vi "Write Sample Push.Sample mBar.vi"(6 "Publish (T)":bool=TRUE, 8 "error in (no error)":errorcluster, 10 "Sample mBar (0)":dbl, 11 "cRIO-CO2 in":refnum<class "cRIO-CO2.lvclass">) -> (0 "error out":errorcluster, 3 "cRIO-CO2 out":refnum<class "cRIO-CO2.lvclass">)   [LabVIEW 2015, in "cRIO-Carbondioxide.lvlib" / "cRIO-CO2.lvlib" / "cRIO-CO2.lvclass"]
uses:
  cRIO-CO2.lvclass
  cRIO-CO2.lvclass/cRIO-CO2.ctl
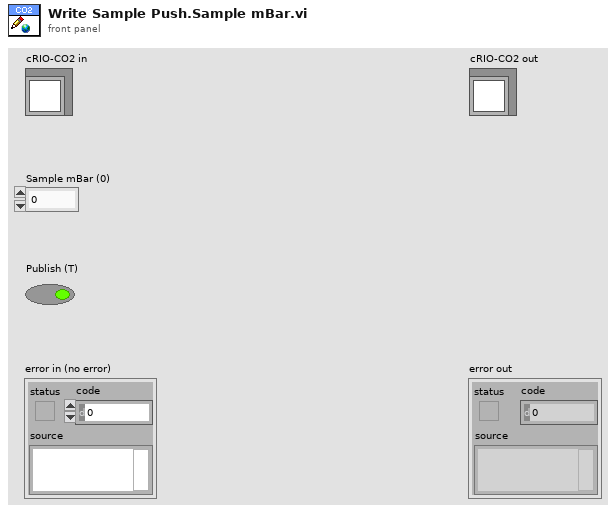
[diagram p1: front panel]
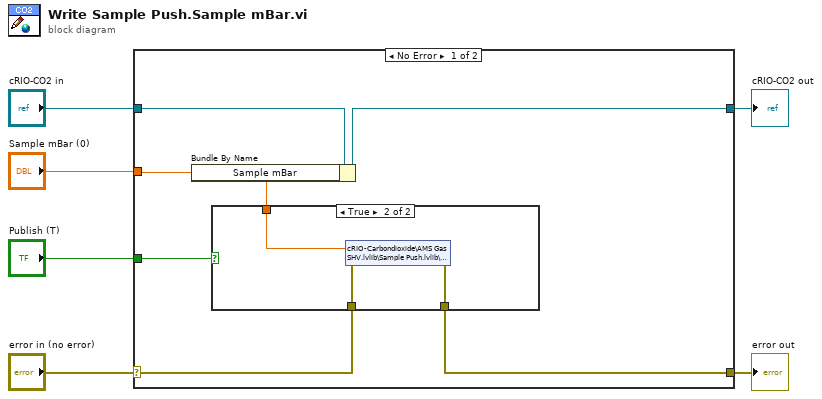
[diagram p0: block diagram]
diagram:
  n1 = case shown="No Error" "error in (no error)" {
    selector: "error in (no error)" -> [w8 w18]
    tunnel: [w7 w18] -> w5
    tunnel: [w11 w17] -> w3
    tunnel: "cRIO-CO2 in" -> [w12 w17]
    tunnel: "Publish (T)" -> [w9 _]
    tunnel: "Sample mBar (0)" -> [w10 _]
    frame No Error {
      n2 = Bundle By Name(cluster=w12, "Sample mBar"=w10) -> (w11:refnum<class "cRIO-CO2.lvclass">)
      n3 = case shown="True" w9 {
        tunnel: w10 -> [_ w14]
        tunnel: w8 -> [w13 w16]
        tunnel: [w13 w15] -> w7
        frame False {
        }
        frame True {
          n4 = shared-variable "cRIO-Carbondioxide\\AMS Gas SHV.lvlib\\Sample Push.lvlib\\Initial mBar"(w14, error in=w16) -> (error out=w15:errorcluster)
        }
      }
    }
    frame Error {
    }
  }
  "error out" <- w5
  "cRIO-CO2 out" <- w3
